vi "GlobalVisionVars.vi"() -> ()   [LabVIEW 2015]
panel:
  out "SettleCounter":dbl
  out "TargetDistance":dbl
  out "NumberOfParticles":i32
  out "TargetRight":bool
  out "TargetLeft":bool
  out "OnTarget":bool
  out "Heading":dbl
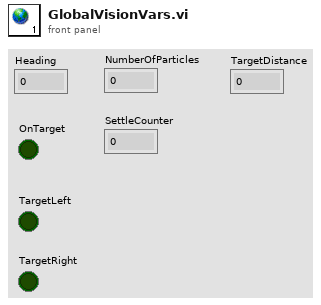
[diagram p1: front panel]
diagram:
